vi "DAQ_PWM.vi"() -> ()   [LabVIEW 2020]
panel:
  in  "Slide":dbl(slide) scale=1.0..2.0
  in  "Offset":dbl
  in  "Amplitude":dbl=1.65
  in  "stop":bool
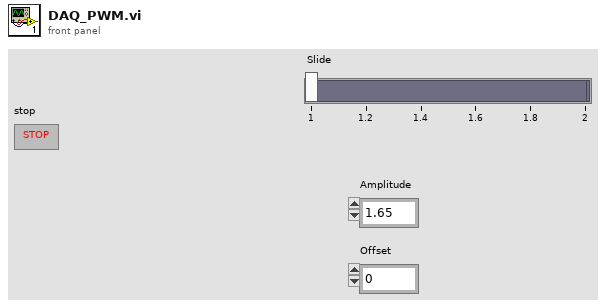
[diagram p1: front panel]
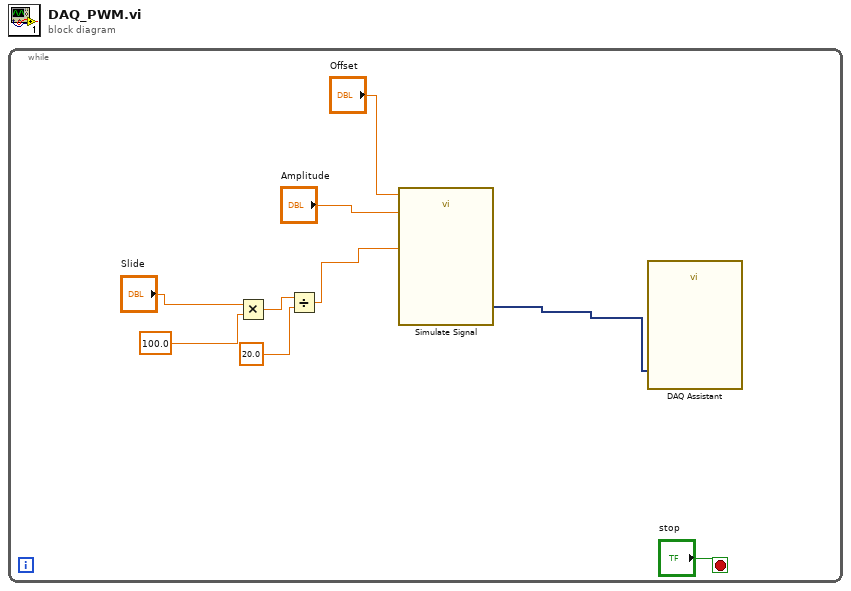
[diagram p0: block diagram]
diagram:
  n1 = while {
    stop <- "stop" stop-if-true
    n2 = Multiply(x="Slide", y=100.0) -> (x*y=w3:dbl)
    n3 = Divide(x=w3, y=20.0) -> (x/y=w1:dbl)
    n4 = call "Simulate Signal"("Offset"="Offset", "Duty Cycle (%)"=w1, "Amplitude"="Amplitude") -> ("Square"=w6:dynamicdata)  [unwired: 11 in, 1 out]
    n5 = call "DAQ Assistant"("data"=w6) -> ()  [unwired: 17 in, 2 out]
  }
